vi "Generation Engine.vi"(0 "synchronous start trigger":bool, 1 "reset":bool, 5 "sw start trigger":bool, 7 "stop trigger in":bool, 9 "packet timing error detected":bool, 11 "generation done":bool, 12 "ready for start trigger":bool) -> (4 "generation state":T1, 6 "start":bool, 8 "stop":bool)   [LabVIEW 2020, in "GettingStarted_Gen_148X_FPGA.lvlib"]
uses:
  GettingStarted_Gen_148X_FPGA.lvlib
  <instrlib>/FlexRIO/CSI-2/v2/FPGA/Types/Generation Engine State.ctl
  <instrlib>/FlexRIO/CSI-2/v2/FPGA/NI CSI-2 API FPGA v2.lvlib
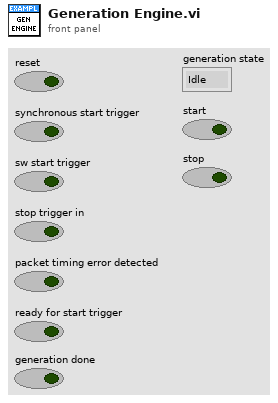
[diagram p1: front panel]
types:
  T1 = typedef "NI CSI-2 API FPGA v2.lvlib/Generation Engine State.ctl" = enum8{"Idle", "Ready For Start Trigger", "Generate Packets", "Done", "Error"}
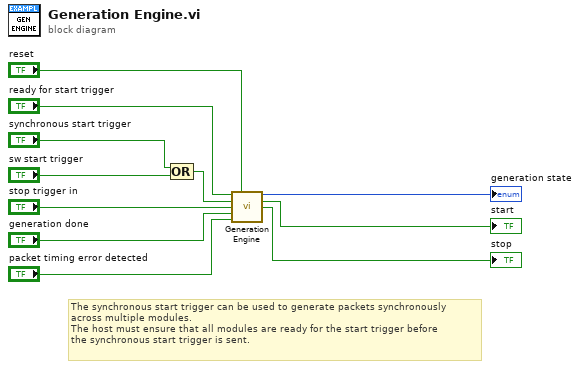
[diagram p0: block diagram]
diagram:
  # "The synchronous start trigger can be used to generate packets synchronously \nacross multiple modules. \nThe host must ensure that all modules are ready for the start trigger before \nthe synchronous start trigger is sent."
  n1 = Compound Arithmetic op=OR("synchronous start trigger", "sw start trigger") -> (w1:bool)
  n2 = call <instrlib>:"Generation Engine.vi"("ready for start trigger"="ready for start trigger", "reset"="reset", "start trigger"=w1, "stop trigger"="stop trigger in", "generation done"="generation done", "error"="packet timing error detected") -> ("state"=→"generation state":T1, "start"=→"start":bool, "stop"=→"stop":bool)  [unwired: 7 in]
